vi "Silenceable Continue Dialog.vi"(6 "window title":string="Alert", 7 "config key":string="NI.SilenceDialog", 8 "error in (no error)":errorcluster, 11 "message in":string) -> (0 "error out":errorcluster, 1 "Cancelled?":bool)   [LabVIEW 2020]
doc: "This VI presents a dialog to the user that allows them to continue or cancel an operation. The dialog includes a \"Do not show this decision again\" checkbox. If user chooses to cancel the operation, this setting is not remembered. If the user continues the operation, the state of the checkbox is remembered in the LabVIEW or built application configuration file. If true, the dialog will not be seen in the future and the operation will be assumed to continue."
uses:
  <resource>/dialog/lvconfig.llb/LV Config Read Boolean.vi
  <resource>/dialog/lvconfig.llb/LV Config Write Boolean.vi
panel:
  in  "error message":string="The config key cannot be an empty string."
  out "message":string
  in  "Do not show this decision again":bool
  in  "Cancel":bool
  in  "Continue":bool
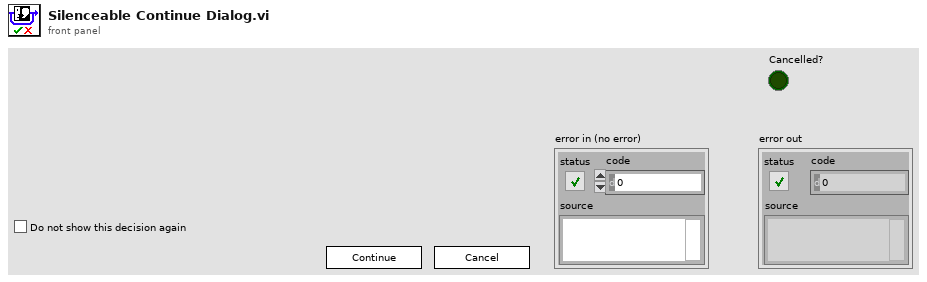
[diagram p1: front panel]
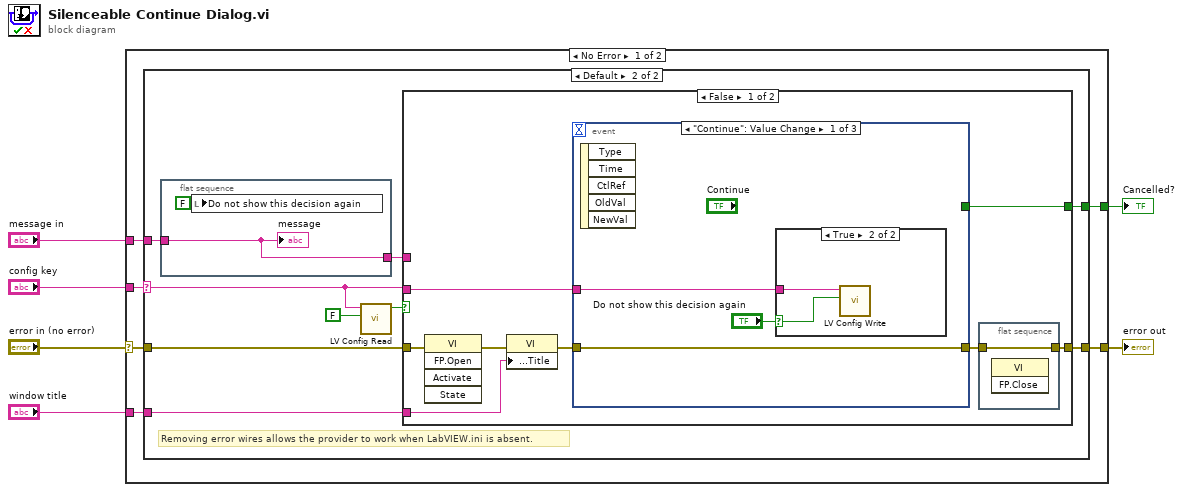
[diagram p0: block diagram]
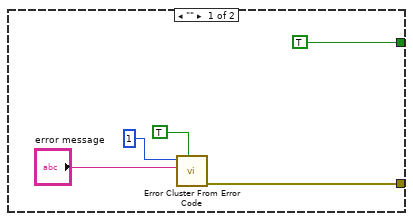
[diagram p2: hidden frame]
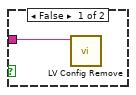
[diagram p3: hidden frame]
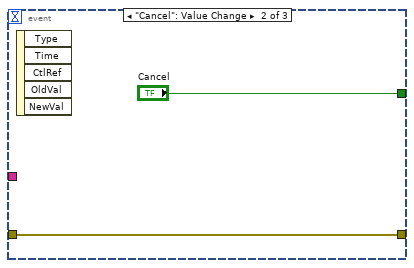
[diagram p4: hidden frame]
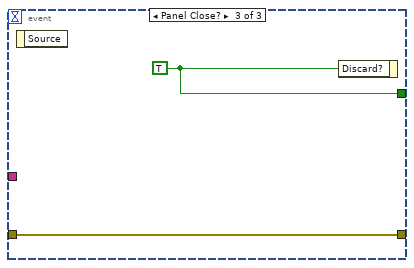
[diagram p5: hidden frame]
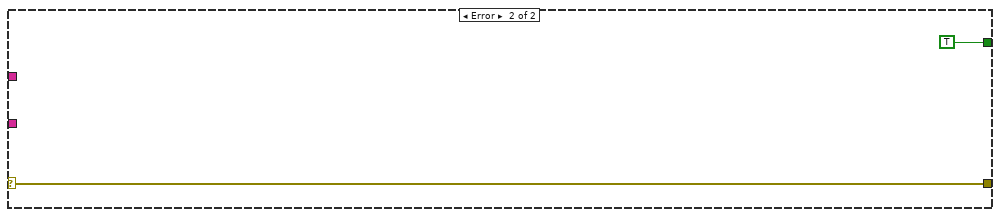
[diagram p7: hidden frame]
diagram:
  n1 = case shown="No Error" "error in (no error)" {
    selector: "error in (no error)" -> [w10 w49]
    tunnel: [w12 TRUE ("Discard?")] -> w6
    tunnel: [w11 w49] -> w4
    tunnel: "config key" -> [w9 _]
    tunnel: "window title" -> [w8 _]
    tunnel: "message in" -> [w7 _]
    frame No Error {
      n2 = case shown="Default" w9 {
        selector: w9 -> [_ w21]
        tunnel: [TRUE ("Discard?") w26] -> w12
        tunnel: [w14 w23] -> w11
        tunnel: w10 -> [_ w22]
        tunnel: w8 -> [_ w19]
        tunnel: w7 -> [_ w18]
        frame "" {
          n3 = call <vilib>:"Error Cluster From Error Code.vi"("show call chain? (False)"=TRUE, "error message (\"\")"="error message", "error code (0)"=1) -> ("error out"=w14:errorcluster)  [unwired: 6 in]
        }
        frame Default {
          # "Removing error wires allows the provider to work when LabVIEW.ini is absent."
          n4 = flat-sequence {
            tunnel: [w27] -> w20
            tunnel: w18 -> [w27]
            frame #0 {
              n5 = local write "Do not show this decision again"(FALSE ("Don't show this dialog again.")) -> ()
              "message" <- w27
            }
          }
          n6 = call-poly <resource>:"LV Config Read.vi"("default value"=FALSE ("Use Reference Method"), "key"=w21) -> ("value"=w24:bool)  [unwired: 3 in, 2 out]
          n7 = case shown="False" w24 {
            tunnel: [w36 _] -> w26
            tunnel: w21 -> [w35 _]
            tunnel: w22 -> [w34 w48]
            tunnel: [w30 w48] -> w23
            tunnel: w20 -> [_ _]
            tunnel: w19 -> [w31 _]
            frame False {
              n8 = invoke class="VI" method="FP.Open"(error in=w34) -> (error out=w33:errorcluster)  [unwired: 4 in, 4 out]
              n9 = property class="VI"(error in=w33, "Front Panel.Title"=w31) -> (error out=w32:errorcluster)  [unwired: 1 in, 1 out]
              n10 = event shown="[0] \"Continue\": Value Change" {
                selector: _ -> [_ _ _]
                dyn-events: _ -> [_ _ _]
                timeout: _ -> [_ _ _]
                tunnel: [_ "Cancel" w47] -> w36
                tunnel: w35 -> [w40 _ _]
                tunnel: w32 -> [w38 w44 w46]
                tunnel: [w38 w44 w46] -> w29
                event "Continue": Value Change {
                  n11 = event-data() -> ()  [unwired: 1 in, 5 out]
                  n12 = case shown="True" "Do not show this decision again" {
                    selector: "Do not show this decision again" -> [_ w42]
                    tunnel: w40 -> [w41 w43]
                    frame False {
                      n13 = call <resource>:"LV Config Remove.vi"("key"=w41) -> ()  [unwired: 6 in, 1 out]
                    }
                    frame True {
                      n14 = call-poly <resource>:"LV Config Write.vi"("value"=w42, "key"=w43) -> ()  [unwired: 5 in, 1 out]
                    }
                  }
                }
                event "Cancel": Value Change {
                  n15 = event-data() -> ()  [unwired: 1 in, 5 out]
                }
                event Panel Close? {
                  w47 = TRUE ("Discard?")
                  n16 = event-data() -> ()  [unwired: 1 in, 1 out]
                  n17 = event-data("Discard?"=w47) -> ()  [unwired: 1 in, 1 out]
                }
              }
              n18 = flat-sequence {
                tunnel: [w37] -> w30
                tunnel: w29 -> [w37]
                frame #0 {
                  n19 = invoke class="VI" method="FP.Close"() -> ()  [unwired: 3 in, 3 out]
                }
              }
            }
            frame True {
            }
          }
        }
      }
    }
    frame Error {
    }
  }
  "Cancelled?" <- w6
  "error out" <- w4
